vi "WaitForInitDone.vi"(2 "error in (no error)":errorcluster, 3 "Preferences.lvclass":refnum<class "SetListPrefs.lvclass">) -> (0 "error out":errorcluster, 1 "Preferences out":refnum<class "SetListPrefs.lvclass">)   [LabVIEW 2013, in "SetListPrefs.lvclass"]
uses:
  SetListPrefs.lvclass
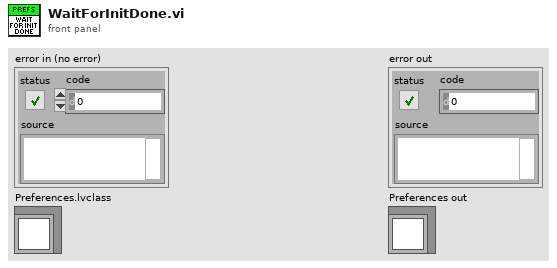
[diagram p1: front panel]
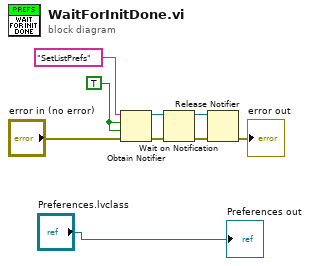
[diagram p0: block diagram]
diagram:
  w8 = TRUE
  n1 = Obtain Notifier(name (unnamed)="SetListPrefs", notification data type=w8, create if not found? (T)=w8, error in (no error)="error in (no error)") -> (notifier out=w5:refnum<notifier>, error out=w6:errorcluster)  [unwired: 1 out]
  n2 = Wait on Notification(notifier=w5, error in (no error)=w6) -> (notifier out=w3:refnum<notifier>, error out=w4:errorcluster)  [unwired: 2 in, 2 out]
  n3 = Release Notifier(notifier=w3, error in (no error)=w4) -> (error out=→"error out":errorcluster)  [unwired: 1 in, 2 out]
  "Preferences out" <- "Preferences.lvclass"
